vi "Multiclamp Test Signal.vi"(0 "Handler":i32, 1 "set":bool, 9 "pnErrorIn":i32, 11 "error in (no error)":errorcluster, 12 "Frequency":dbl(ring)=100.0 items=["2 Hz"=2.0, "5 Hz"=5.0, "10 Hz"=10.0, "20 Hz"=20.0, "50 Hz"=50.0, "60 Hz"=60.0, "100 Hz"=100.0, "200 Hz"=200.0, "500 Hz"=500.0, "1000 Hz"=1000.0], 13 "Amplitude [mV]":i32=10 min=-1000 max=1000 format="%#.0f") -> (4 "Handler":i32, 10 "pnError out":i32, 15 "error out":errorcluster)   [LabVIEW 2012, in "MultiClamp 700B Controls.lvlib"]
uses:
  MultiClamp 700B Controls.lvlib
  AxMultiClampMsg/AxMultiClampMsg.lvlib
panel:
  in  "Tab Control":enum32{"Page 1", "Page 2"}(tab)
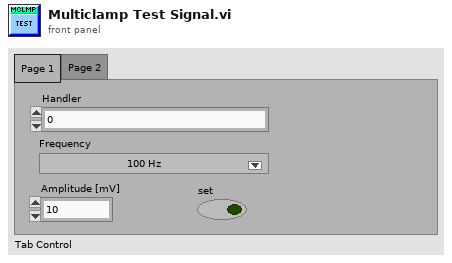
[diagram p1: front panel]
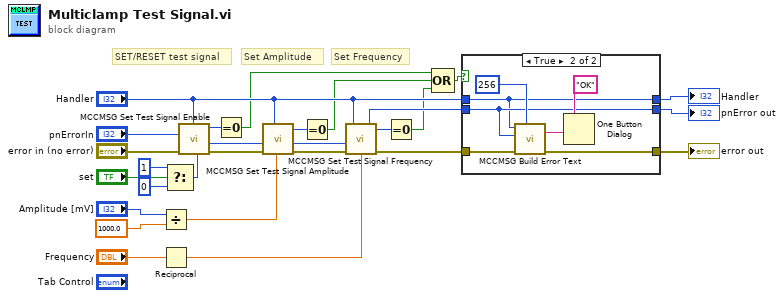
[diagram p0: block diagram]
diagram:
  # "SET/RESET test signal"
  # "Set Frequency"
  # "Set Amplitude"
  n1 = Divide(x="Amplitude [mV]", y=1000.0) -> (x/y=w3:dbl)
  n2 = Reciprocal(x="Frequency") -> (1/x=w28:dbl)
  n3 = Select(t=1, s="set", f=0) -> (s? t:f=w20:i32)
  n4 = call "MCCMSG Set Test Signal Enable.vi"("error in (no error)"="error in (no error)", "pnError"="pnErrorIn", "bEnable"=w20, "hMCCmsg"="Handler") -> ("error out"=w16:errorcluster, "pnError out"=w15:i32, "function return"=w10:i32)  [unwired: 5 in]
  n5 = Equal To 0?(x=w10) -> (x = 0?=w7:bool)
  n6 = call "MCCMSG Set Test Signal Amplitude.vi"("error in (no error)"=w16, "pnError"=w15, "dAmplitude"=w3, "hMCCmsg"="Handler") -> ("error out"=w14:errorcluster, "pnError out"=w13:i32, "function return"=w11:i32)  [unwired: 5 in]
  n7 = Equal To 0?(x=w11) -> (x = 0?=w8:bool)
  n8 = call "MCCMSG Set Test Signal Frequency.vi"("error in (no error)"=w14, "pnError"=w13, "dFrequency"=w28, "hMCCmsg"="Handler") -> ("error out"=w24:errorcluster, "pnError out"=w26:i32, "function return"=w25:i32)  [unwired: 5 in]
  n9 = Equal To 0?(x=w25) -> (x = 0?=w9:bool)
  n10 = Compound Arithmetic op=OR(w7, w8, w9) -> (w6:bool)
  n11 = case shown="True" w6 {
    tunnel: w26 -> [w31 w34]
    tunnel: w24 -> [w29 w38]
    tunnel: "Handler" -> [w30 w33]
    tunnel: [w31 w34] -> w17
    tunnel: [w30 w33] -> w18
    tunnel: [w29 w32] -> w19
    frame False {
    }
    frame True {
      n12 = call "MCCMSG Build Error Text.vi"("uMaxLen"=u32 256, "error in (no error)"=w38, "nErrorNum"=w34, "hMCCmsg"=w33) -> ("error out"=w32:errorcluster, "sTxtBuf out"=w37:string)  [unwired: 5 in, 1 out]
      n13 = One Button Dialog(message=w37, button name ("OK")="OK") -> ()  [unwired: 1 out]
    }
  }
  "error out" <- w19
  "Handler" <- w18
  "pnError out" <- w17
